vi "RPTID Declare Notifier.vi"(8 "error in":errorcluster, 11 "RPTID Data":T1[](array[typedef])) -> (0 "error out":errorcluster, 3 "RPTID Notifier":refnum<notifier>[](array[refnum]))   [LabVIEW 2020, in "SECS Communication.lvlib" / "SECS Data Class.lvclass"]
uses:
  SECS Data Class.lvclass
  RPTID Data.ctl
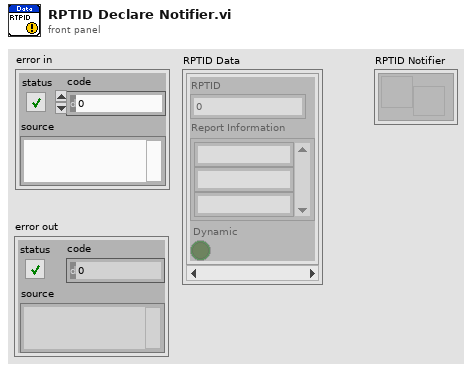
[diagram p1: front panel]
types:
  T1 = typedef "SECS Communication.lvlib/SECS Data Class.lvclass/RPTID Data.ctl" = cluster{"RPTID":u32, "Report Information":string[], "Dynamic":bool}
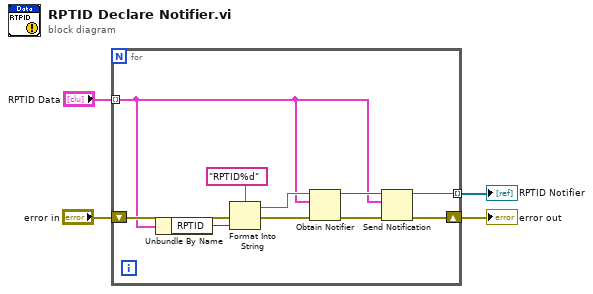
[diagram p0: block diagram]
diagram:
  n1 = for {
    tunnel: "RPTID Data" -> [w7] mode=indexing
    shift-right: [w6] -> w2
    shift-left: "error in" -> [w14]
    tunnel: [w5] -> w1 mode=indexing
    n2 = Unbundle By Name(w7) -> ("RPTID"=w13:u32)
    n3 = Format Into String(format string="RPTID%d", error in=w14, w13) -> (resulting string=w10:string, error out=w11:errorcluster)  [unwired: 1 in]
    n4 = Obtain Notifier(name (unnamed)=w10, notification data type=w7, error in (no error)=w11) -> (notifier out=w9:refnum<notifier>, error out=w8:errorcluster)  [unwired: 1 in, 1 out]
    n5 = Send Notification(notification=w7, notifier=w9, error in (no error)=w8) -> (notifier out=w5:refnum<notifier>, error out=w6:errorcluster)
  }
  "error out" <- w2
  "RPTID Notifier" <- w1
